vi "FIRE CONTROL.vi"(8 "error in (no error)":errorcluster, 11 "control\ncluster":T2) -> (0 "error out":errorcluster, 3 "control\ncluster out":T2)   [LabVIEW 2023]
uses:
  ctrl defs/ctrl controllers.ctl
  ctrl defs/ctrl Xbox-buttons.ctl
  Global stack names.vi
panel:
  in  "button for\nFLAP":T1=enum."RB"
  in  "button for\nAMP SPEED":T1=enum."Y"
  in  "button for\nFIRE":T1
  in  "button for\nPUKE":T1=enum."B"
  in  "button for\nINTAKE":T1=enum."X"
  in  "notes":string="Joystick 1- co-pilot\n\nINTAKE toggles intake rollers\n\nPUKE reverses intake & clears NOTE flag; timed to shut off\n\nFIRE starts firing sequence\n\nAMP SPEED slows shooter speed\n\nFLAP toggles flap/bumper extension"
  out "Buttons":bool[](array[boolean])
  out "POVs":i16[](array[numeric])
  out "Axes":dbl[](array[numeric])
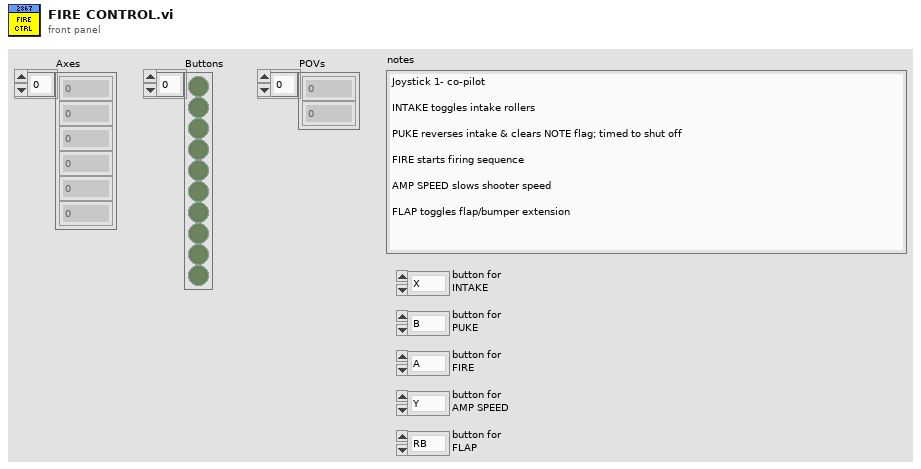
[diagram p1: front panel]
types:
  T1 = typedef "ctrl Xbox-buttons.ctl" = enum16{"A", "B", "X", "Y", "LB", "RB", "Back", "Start", "LJ", "RJ"}
  T2 = typedef "ctrl controllers.ctl" = cluster{"Axes":dbl[], "Buttons":bool[], "POVs":i16[]}
  T3 = typedef "ctrl stack - INTAKE SHOOTER.ctl" = cluster{"INTAKE STATE":string, "RUN INTAKE?":string, "RUN REVERSE?":string, "NOTE LOADED?":string, "SHOOTER STATE":string, "SHOOTER FIRE?":string, "SHOOT AMP?":string, "EXTEND FLAP?":string, "LOOKING for NOTE":string, "OVERIDE NOTE CHECK":string}
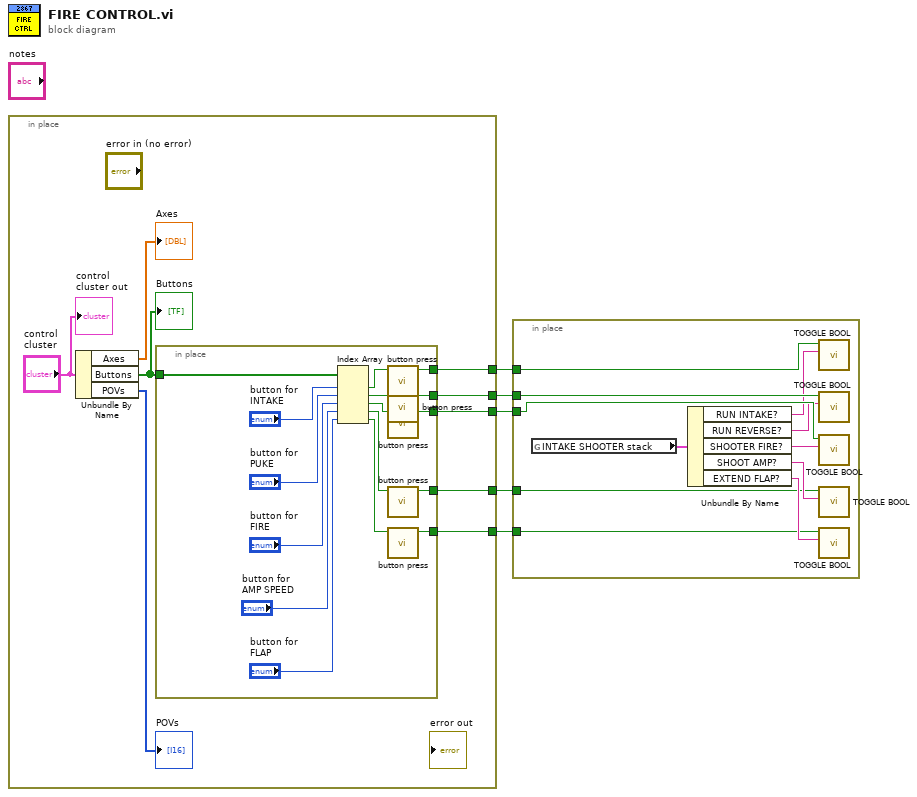
[diagram p0: block diagram]
diagram:
  n1 = in-place {
    in-place-border: [w10] -> w2
    in-place-border: [w9] -> w3
    in-place-border: [w8] -> w4
    in-place-border: [w7] -> w5
    in-place-border: [w6] -> w1
    n2 = Unbundle By Name("control\ncluster") -> ("Axes"=→"Axes":dbl[], "Buttons"=w11:bool[], "POVs"=→"POVs":i16[])
    "Buttons" <- w11
    n3 = in-place {
      in-place-border: w11 -> [w30]
      in-place-border: [w27] -> w10
      in-place-border: [w25] -> w9
      in-place-border: [w23] -> w8
      in-place-border: [w18] -> w7
      in-place-border: [w15] -> w6
      n4 = Index Array(array=w30, index #1="button for\nINTAKE", index #2="button for\nPUKE", index #3="button for\nFIRE", index #4="button for\nAMP SPEED", index #5="button for\nFLAP") -> (element #1=w29:bool, element #2=w26:bool, element #3=w24:bool, element #4=w19:bool, element #5=w16:bool)
      n5 = call "button press.vi"("button IN"=w29) -> ("Button Pressed?"=w27:bool)  [unwired: 10 in]
      n6 = call "button press.vi"("button IN"=w26) -> ("Button Pressed?"=w25:bool)  [unwired: 10 in]
      n7 = call "button press.vi"("button IN"=w24) -> ("Button Pressed?"=w23:bool)  [unwired: 10 in]
      n8 = call "button press.vi"("button IN"=w19) -> ("Button Pressed?"=w18:bool)  [unwired: 10 in]
      n9 = call "button press.vi"("button IN"=w16) -> ("Button Pressed?"=w15:bool)  [unwired: 10 in]
    }
    "control\ncluster out" <- "control\ncluster"
  }
  n10 = in-place {
    in-place-border: w5 -> [w32]
    in-place-border: w4 -> [w38]
    in-place-border: w3 -> [w37]
    in-place-border: w2 -> [w35]
    in-place-border: w1 -> [w31]
    n11 = global read "Global stack names.vi" "INTAKE SHOOTER stack"() -> (w41:T3)
    n12 = Unbundle By Name(w41) -> ("RUN INTAKE?"=w34:string, "RUN REVERSE?"=w36:string, "SHOOTER FIRE?"=w39:string, "SHOOT AMP?"=w40:string, "EXTEND FLAP?"=w33:string)
    n13 = call "TOGGLE BOOL.vi"("stack ref name"=w34, "Button Pressed?"=w35) -> ()  [unwired: 9 in, 1 out]
    n14 = call "TOGGLE BOOL.vi"("stack ref name"=w36, "Button Pressed?"=w37) -> ()  [unwired: 9 in, 1 out]
    n15 = call "TOGGLE BOOL.vi"("stack ref name"=w39, "Button Pressed?"=w38) -> ()  [unwired: 9 in, 1 out]
    n16 = call "TOGGLE BOOL.vi"("stack ref name"=w40, "Button Pressed?"=w32) -> ()  [unwired: 9 in, 1 out]
    n17 = call "TOGGLE BOOL.vi"("stack ref name"=w33, "Button Pressed?"=w31) -> ()  [unwired: 9 in, 1 out]
  }
